vi "Make Sensor String.vi"(8 "error in (no error)":errorcluster, 10 "Sensor?":bool) -> (0 "error out":errorcluster, 2 "Sensor string":string)   [LabVIEW 2012]
doc: "Creates the required zoom string."
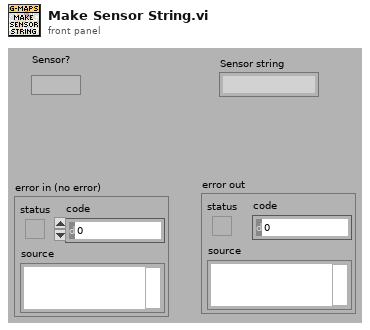
[diagram p1: front panel]
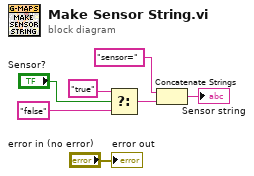
[diagram p0: block diagram]
diagram:
  n1 = Select(t="true" ("URL"), s="Sensor?", f="false" ("URL")) -> (s? t:f=w1:string)
  n2 = Concatenate Strings("sensor=" ("URL"), w1) -> (→"Sensor string":string)
  "error out" <- "error in (no error)"
